vi "Test TS Environment Manager - Cache File Exists.vi"() -> (0 "error out":errorcluster)   [LabVIEW 2025]
doc: "Tests setting up of an existing cache file."
uses:
  <userlib>/_OpenG.lib/file/file.llb/File Exists - Scalar__ogtk.vi
  <vilib>/Utility/config.llb/Write Key (Path).vi
  <userlib>/_OpenG.lib/file/file.llb/openg_file.lvlib
  <vilib>/addons/_JKI Toolkits/Caraya/classes/Test/Test.lvclass
  src/Libraries/TS Environment Manager/TS Environment Manager.lvlib
  <vilib>/Utility/config.llb/NI_LVConfig.lvlib
  <vilib>/addons/_JKI Toolkits/Caraya/classes/Assert/Assert.lvclass
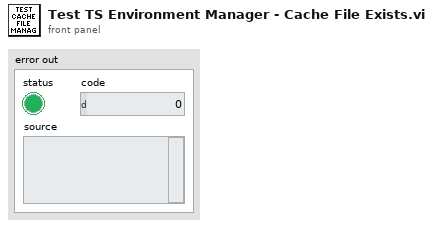
[diagram p1: front panel]
types:
  T1 = typedef "NI_LVConfig.lvlib/Config Data RefNum.ctl" = refnum<k1>
  T2 = typedef "Profile--cluster.ctl" = cluster{"Name":string, "Version":string, "Architecture":T3, "Environment":path}
  T3 = typedef "Architecture--enum.ctl" = enum16{"32bit", "64bit"}
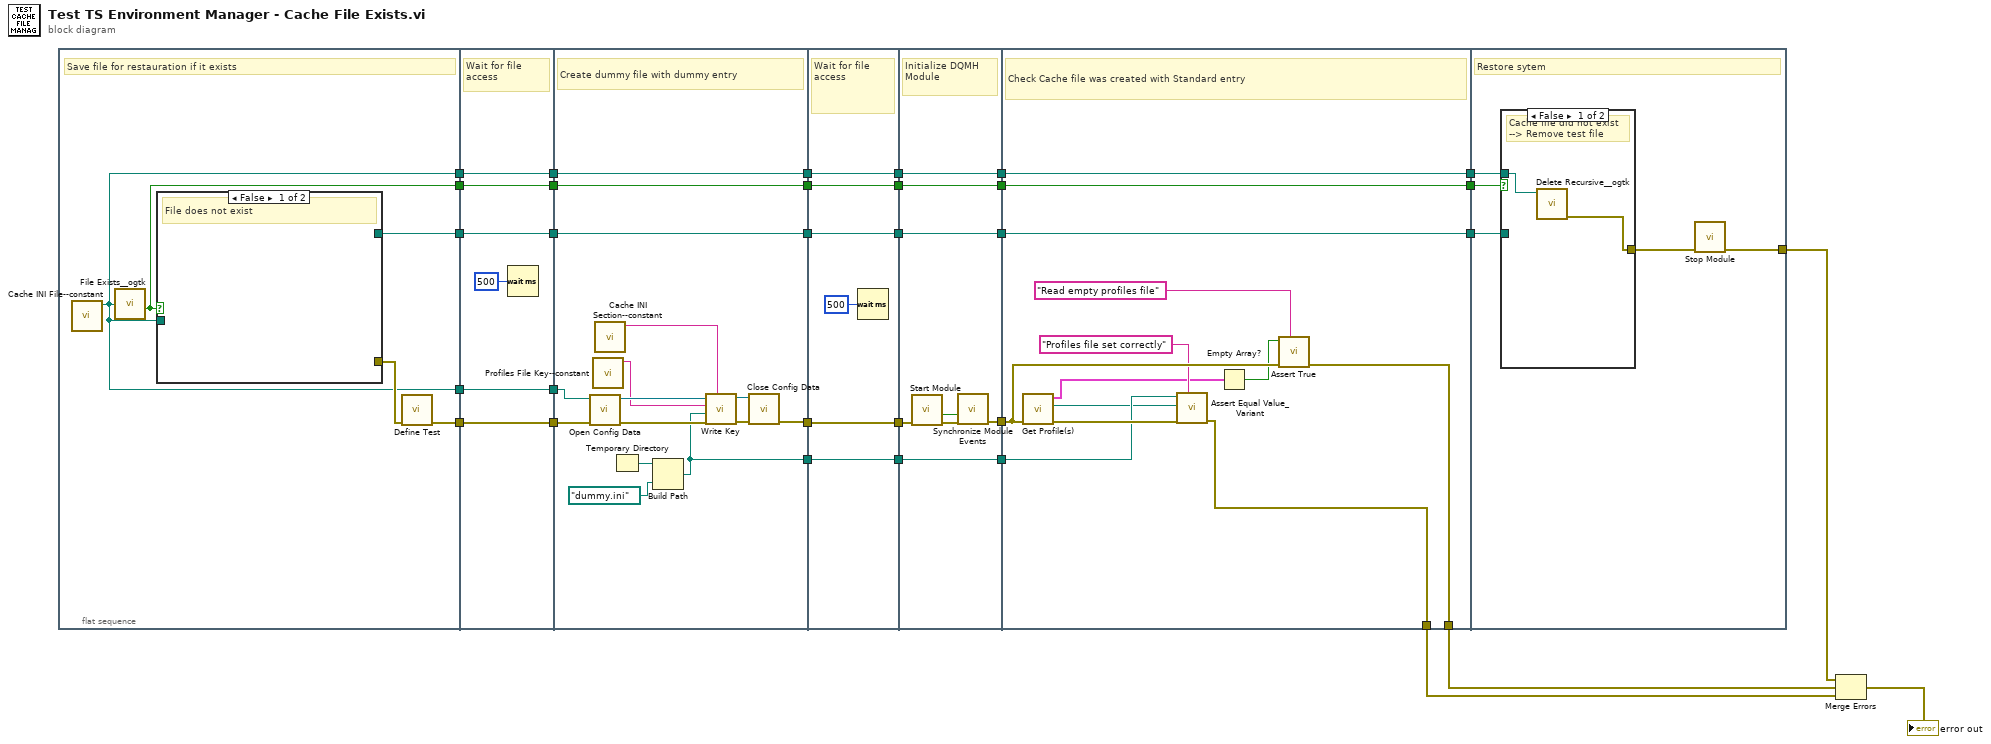
[diagram p0: block diagram]
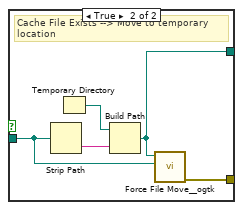
[diagram p2: hidden frame]
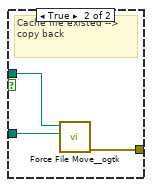
[diagram p3: hidden frame]
diagram:
  n1 = flat-sequence {
    tunnel: [w37] -> w32
    tunnel: [w33] -> w22
    tunnel: [w35] -> w18
    tunnel: [w34] -> w14
    tunnel: [w33] -> w10
    tunnel: w32 -> [w48]
    tunnel: [w48] -> w31
    tunnel: [w46] -> w23
    tunnel: w22 -> [w46]
    tunnel: [w45] -> w19
    tunnel: w18 -> [w45]
    tunnel: [w44] -> w15
    tunnel: w14 -> [w44]
    tunnel: [w43] -> w11
    tunnel: w10 -> [w43]
    tunnel: w31 -> [w61]
    tunnel: w23 -> [w52]
    tunnel: [w60] -> w25
    tunnel: [w59] -> w9
    tunnel: w19 -> [w59]
    tunnel: [w58] -> w7
    tunnel: w15 -> [w58]
    tunnel: [w57] -> w5
    tunnel: w11 -> [w57]
    tunnel: [w49] -> w1
    tunnel: w25 -> [w69]
    tunnel: [w69] -> w24
    tunnel: w9 -> [w68]
    tunnel: [w68] -> w8
    tunnel: w7 -> [w67]
    tunnel: [w67] -> w6
    tunnel: w5 -> [w66]
    tunnel: [w66] -> w4
    tunnel: [w64] -> w2
    tunnel: w1 -> [w64]
    tunnel: w24 -> [w76]
    tunnel: [w75] -> w30
    tunnel: [w73] -> w20
    tunnel: w8 -> [w73]
    tunnel: [w72] -> w16
    tunnel: w6 -> [w72]
    tunnel: [w71] -> w12
    tunnel: w4 -> [w71]
    tunnel: [w70] -> w3
    tunnel: w2 -> [w70]
    tunnel: [w89] -> w29
    tunnel: [w88] -> w28
    tunnel: [w86] -> w21
    tunnel: [w85] -> w17
    tunnel: [w84] -> w13
    tunnel: w12 -> [w84]
    tunnel: w16 -> [w85]
    tunnel: w20 -> [w86]
    tunnel: w30 -> [w87]
    tunnel: w3 -> [w83]
    tunnel: w21 -> [w93]
    tunnel: w17 -> [w92]
    tunnel: w13 -> [w91]
    tunnel: [w94] -> w26
    frame #0 {
      # "Save file for restauration if it exists"
      n2 = call "Cache INI File--constant.vi"() -> ("Cache INI File"=w33:path)  [unwired: 11 in]
      n3 = call-poly <userlib>:"File Exists__ogtk.vi"("file path"=w33) -> ("exists"=w35:bool)  [unwired: 6 in, 1 out]
      n4 = case shown="False" w35 {
        tunnel: w33 -> [_ w39]
        tunnel: [_ w38] -> w34
        tunnel: [_ w42] -> w36
        frame False {
          # "File does not exist"
        }
        frame True {
          # "Cache File Exists --> Move to temporary location"
          n5 = Strip Path(path=w39) -> (name=w40:string)  [unwired: 1 out]
          n6 = Temporary Directory() -> (w41:path)
          n7 = Build Path(base path=w41, name or relative path=w40) -> (appended path=w38:path)
          n8 = call <userlib>:"Force File Move__ogtk.vi"("source"=w39, "target"=w38) -> ("error out"=w42:errorcluster)  [unwired: 4 in, 1 out]
        }
      }
      n9 = call <vilib>:"Define Test.vi"("error in (no error)"=w36) -> ("error out"=w37:errorcluster)  [unwired: 9 in, 1 out]
    }
    frame #1 {
      # "Wait for file access"
      n10 = Wait (ms)(milliseconds to wait=u32 500) -> ()  [unwired: 1 out]
    }
    frame #2 {
      # "Create dummy file with dummy entry"
      n11 = call <vilib>:"Open Config Data.vi"("error in (no error)"=w61, "configuration file path"=w52) -> ("error out"=w63:errorcluster, "refnum"=w56:T1)  [unwired: 7 in, 1 out]
      n12 = call "Profiles File Key--constant.vi"() -> ("Profiles File Key"=w55:string)  [unwired: 11 in]
      n13 = call "Cache INI Section--constant.vi"() -> ("Cache INI Section"=w53:string)  [unwired: 11 in]
      n14 = Temporary Directory() -> (w51:path)
      n15 = Build Path(base path=w51, name or relative path=path "dummy.ini") -> (appended path=w49:path)
      n16 = call-poly <vilib>:"Write Key.vi"("section"=w53, "error in (no error)"=w63, "value"=w49, "key"=w55, "refnum"=w56) -> ("error out"=w62:errorcluster, "refnum out"=w54:T1)  [unwired: 4 in, 1 out]
      n17 = call <vilib>:"Close Config Data.vi"("error in (no error)"=w62, "refnum"=w54) -> ("error out"=w60:errorcluster)  [unwired: 8 in, 1 out]
    }
    frame #3 {
      # "Wait for file access"
      n18 = Wait (ms)(milliseconds to wait=u32 500) -> ()  [unwired: 1 out]
    }
    frame #4 {
      # "Initialize DQMH Module"
      n19 = call "Start Module.vi"("error in"=w76) -> ("error out"=w77:errorcluster, "Wait for Event Sync?"=w74:bool)  [unwired: 6 in, 3 out]
      n20 = call "Synchronize Module Events.vi"("error in"=w77, "Wait for Event Sync?"=w74) -> ("error out"=w75:errorcluster)  [unwired: 9 in]
    }
    frame #5 {
      # "Check Cache file was created with Standard entry"
      n21 = call "Get Profile(s).vi"("error in"=w87) -> ("error out"=w90:errorcluster, "File"=w82:path, "Profile(s)"=w80:T2[])  [unwired: 7 in, 1 out]
      n22 = call <vilib>:"Assert Equal Value_Variant.vi"("Label"="Profiles file set correctly", "error in (no error)"=w90, "Actual"=w82, "Expected"=w83) -> ("error out"=w88:errorcluster)  [unwired: 6 in, 1 out]
      n23 = Empty Array?(array=w80) -> (empty?=w79:bool)
      n24 = call <vilib>:"Assert True.vi"("Label"="Read empty profiles file", "error in (no error)"=w87, "True?"=w79) -> ("error out"=w89:errorcluster)  [unwired: 7 in, 1 out]
    }
    frame #6 {
      # "Restore sytem"
      n25 = case shown="False" w93 {
        tunnel: w92 -> [_ w99]
        tunnel: w91 -> [w96 w98]
        tunnel: [w97 w100] -> w95
        frame False {
          # "Cache file did not exist --> Remove test file"
          n26 = call <userlib>:"Delete Recursive__ogtk.vi"("Path"=w96) -> ("error out"=w97:errorcluster)  [unwired: 9 in, 1 out]
        }
        frame True {
          # "Cache file existed --> copy back"
          n27 = call <userlib>:"Force File Move__ogtk.vi"("source"=w99, "target"=w98) -> ("error out"=w100:errorcluster)  [unwired: 4 in, 1 out]
        }
      }
      n28 = call "Stop Module.vi"("error in"=w95) -> ("error out"=w94:errorcluster)  [unwired: 10 in]
    }
  }
  n29 = Merge Errors(w26, w29, w28) -> (→"error out":errorcluster)
